vi "NotifyOwner(Message).vi"(8 "error in (no error)":errorcluster, 9 "Payload":variant, 10 "Message (empty : payload label)":string, 11 "SMO in":refnum<class "SMO.lvclass">) -> (0 "error out":errorcluster, 3 "SMO out":refnum<class "SMO.lvclass">)   [LabVIEW 2021, in "smo.lvlib" / "SMO.lvclass"]
uses:
  SMO.lvclass
  SMO.lvclass/SMO.ctl
  Support/Attribute.Owner/Attribute.Owner.lvclass
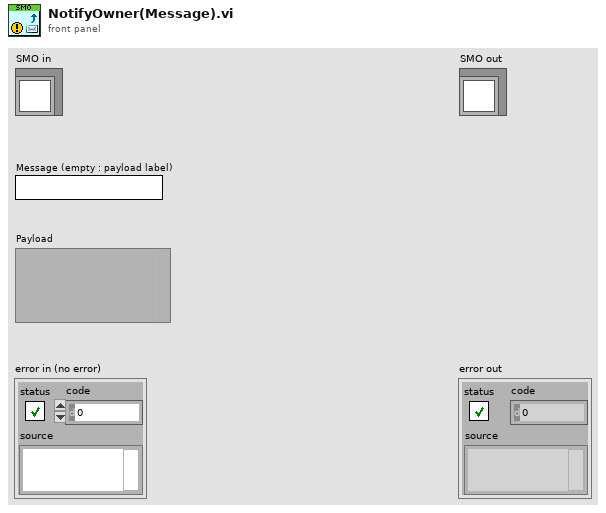
[diagram p1: front panel]
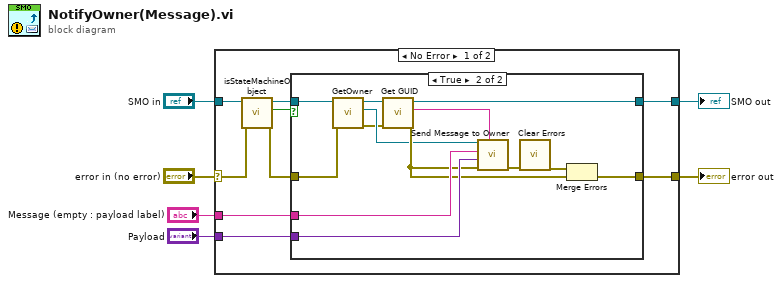
[diagram p0: block diagram]
diagram:
  n1 = case shown="No Error" "error in (no error)" {
    selector: "error in (no error)" -> [w9 w32]
    tunnel: [w15 w32] -> w5
    tunnel: [w14 w31] -> w3
    tunnel: "SMO in" -> [w11 w31]
    tunnel: "Message (empty : payload label)" -> [w13 _]
    tunnel: "Payload" -> [w12 _]
    frame No Error {
      n2 = call "isStateMachineObject.vi"("error in (no error)"=w9, "SMO"=w11) -> ("error out"=w7:errorcluster, "is SMO?"=w8:bool, "SMO out"=w10:refnum<class "SMO.lvclass">)  [unwired: 7 in]
      n3 = case shown="True" w8 {
        tunnel: [w16 w28] -> w15
        tunnel: [w17 w27] -> w14
        tunnel: w13 -> [_ w25]
        tunnel: w12 -> [_ w24]
        tunnel: w10 -> [w17 w19]
        tunnel: w7 -> [w16 w18]
        frame False {
        }
        frame True {
          n4 = call "GetOwner.vi"("error in (no error)"=w18, "SMO in"=w19) -> ("error out"=w20:errorcluster, "Owner"=w22:refnum<class "Attribute.Owner.lvclass">, "SMO out"=w21:refnum<class "SMO.lvclass">)  [unwired: 6 in, 1 out]
          n5 = call "Get GUID.vi"("error in (no error)"=w20, "SMO"=w21) -> ("error out"=w23:errorcluster, "GUID"=w26:string, "SMO out"=w27:refnum<class "SMO.lvclass">)  [unwired: 7 in]
          n6 = call "Send Message to Owner.vi"("GUID"=w26, "error in (no error)"=w23, "Message Payload"=w24, "Message"=w25, "Attribute.Owner in"=w22) -> ("error out"=w30:errorcluster)  [unwired: 5 in, 1 out]
          n7 = call <vilib>:"Clear Errors.vi"("error in (no error)"=w30) -> ("error out"=w29:errorcluster)  [unwired: 5 in, 1 out]
          n8 = Merge Errors(w29, w23) -> (w28:errorcluster)
        }
      }
    }
    frame Error {
    }
  }
  "error out" <- w5
  "SMO out" <- w3
